vi "Check Status.vi"(8 "error in":errorcluster, 11 "connection ID In":refnum<k5>) -> (0 "error out":errorcluster, 2 "Data":string, 3 "connection ID Out":refnum<k5>)   [LabVIEW 2018, in "Labview Python.lvlib"]
uses:
  Labview Python.lvlib
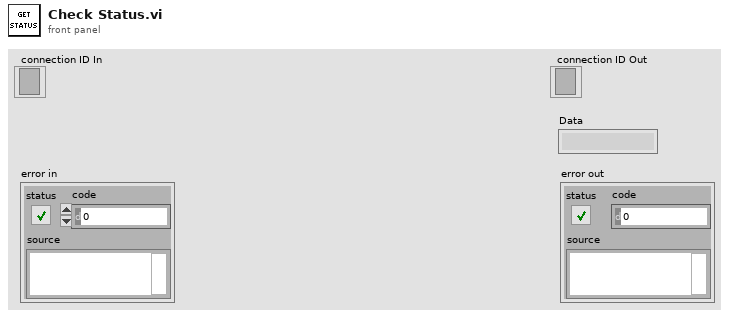
[diagram p1: front panel]
types:
  T1 = enum16{"Standard", "Buffered", "CRLF", "Immediate"}
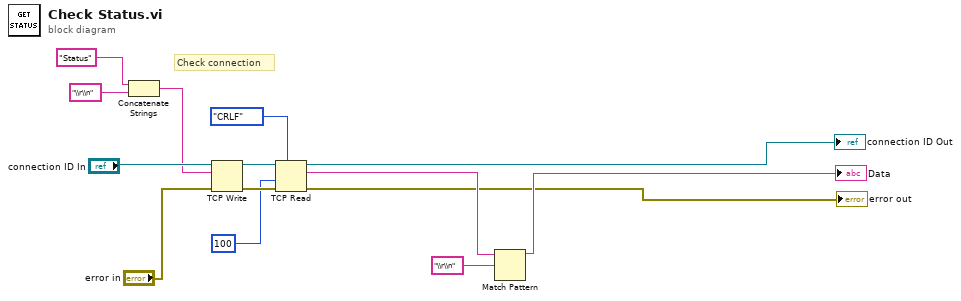
[diagram p0: block diagram]
diagram:
  # "Check connection"
  n1 = Concatenate Strings("Status" ("data in"), "\\r\\n") -> (w10:string)
  n2 = TCP Write(connection ID="connection ID In", data in=w10, error in (no error)="error in") -> (connection ID out=w9:refnum<k5>, error out=w8:errorcluster)  [unwired: 2 out]
  n3 = TCP Read(connection ID=w9, error in (no error)=w8, 7:T1."CRLF" ("mode (standard)"), 9:100 ("timeout ms (25000)")) -> (connection ID out=→"connection ID Out":refnum<k5>, data out=w4:string, error out=→"error out":errorcluster)  [unwired: 1 in]
  n4 = Match Pattern(string=w4, regular expression="\\r\\n") -> (before substring=→"Data":string)  [unwired: 1 in, 3 out]
